vi "Display Console - Show Message.vi"(8 "error in (no error)":errorcluster, 10 "Message Name":T6, 11 "View Model":T1) -> (0 "error out":errorcluster, 2 "Message":string)   [LabVIEW 2017]
doc: "Provides display selected message to user."
uses:
  Controls/Display Console - Message Name.ctl
  View Model/Controls/View Model.ctl
  Error Handler/Controls/Error Model.ctl
  Error Handler/Controls/Error Data.ctl
  Error Handler/Controls/Error Type.ctl
  View Model/Controls/Shared Model.ctl
  Configuration/Controls/Config Model.ctl
  Configuration/Controls/Config CMD.ctl
  Configuration/Controls/Config Data.ctl
  ATM Controller/Controls/Controller Model.ctl
  ATM Controller/Controls/Controller Overhead.ctl
  ATM Controller/Controls/Controller States.ctl
  Controls/Display Console - Message Data.ctl
  User Console View/Controls/User Console - Keypad.ctl
  User Console View/Controls/User Console - Transactions.ctl
  ATM Controller/Controls/Controller CMD.ctl
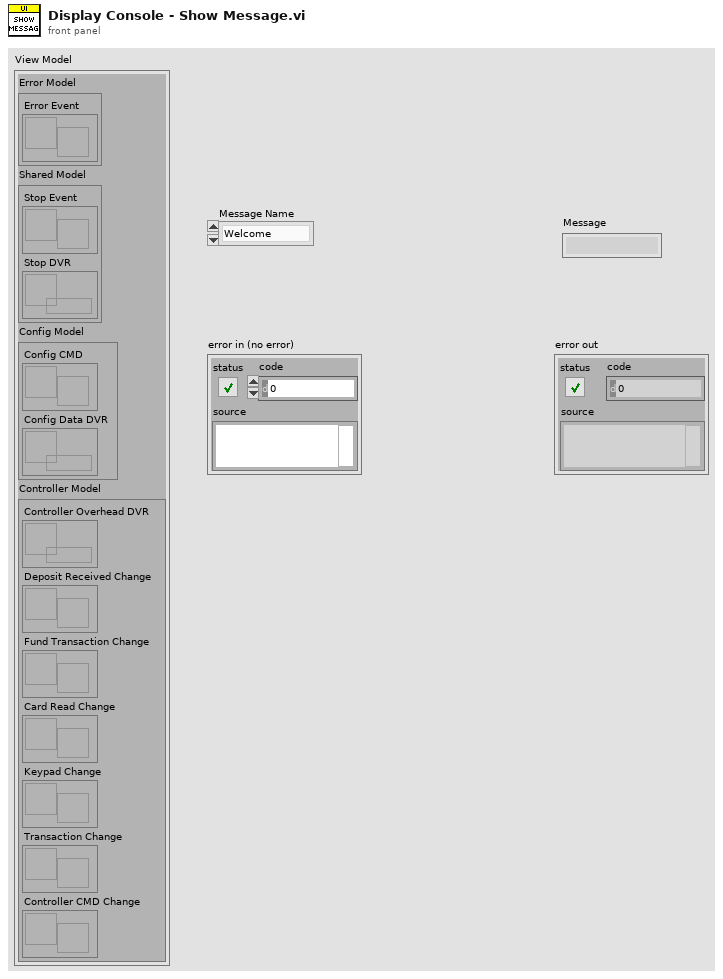
[diagram p1: front panel]
types:
  T1 = typedef "View Model.ctl" = cluster{"Error Model":T2, "Shared Model":T3, "Config Model":T4, "Controller Model":T5}
  T2 = typedef "Error Model.ctl" = cluster{"Error Event":refnum<user-event>}
  T3 = typedef "Shared Model.ctl" = cluster{"Stop Event":refnum<user-event>, "Stop DVR":refnum<data-value>}
  T4 = typedef "Config Model.ctl" = cluster{"Config CMD":refnum<user-event>, "Config Data DVR":refnum<data-value>}
  T5 = typedef "Controller Model.ctl" = cluster{"Controller Overhead DVR":refnum<data-value>, "Deposit Received Change":refnum<user-event>, "Fund Transaction Change":refnum<user-event>, "Card Read Change":refnum<user-event>, "Keypad Change":refnum<user-event>, "Transaction Change":refnum<user-event>, "Controller CMD Change":refnum<user-event>}
  T6 = typedef "Display Console - Message Name.ctl" = enum16{"Welcome", "Idle", "Invalid Login", "Terminate", "Deposit", "Withdrawal", "Fast Cash", "Withdrawal Complete", "Withdrawal Failed", "Balance Inquiry"}
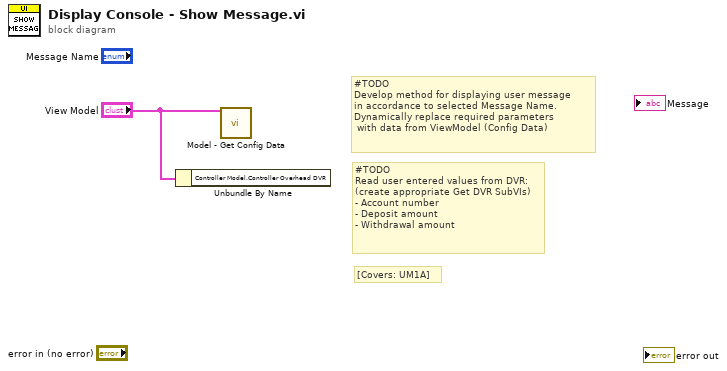
[diagram p0: block diagram]
diagram:
  # "[Covers: UM1A]"
  # "#TODO\nRead user entered values from DVR:\n(create appropriate Get DVR SubVIs)\n- Account number\n- Deposit amount\n- Withdrawal amount"
  # "#TODO\nDevelop method for displaying user message \nin accordance to selected Message Name.\nDynamically replace required parameters\n with data from ViewModel (Config Data)"
  n1 = Unbundle By Name("View Model") -> ()  [unwired: 1 out]
  n2 = call "Model - Get Config Data.vi"("View Model"="View Model") -> ()  [unwired: 8 in, 3 out]
